vi "Boolean Triggers.vi"() -> ()   [LabVIEW 2019]
panel:
  out "Intake":bool
  out "Trigger":bool
  in  "Joystick for Intake":bool
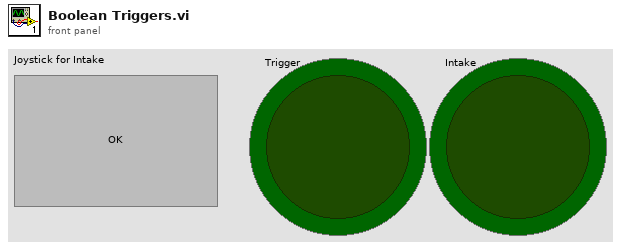
[diagram p1: front panel]
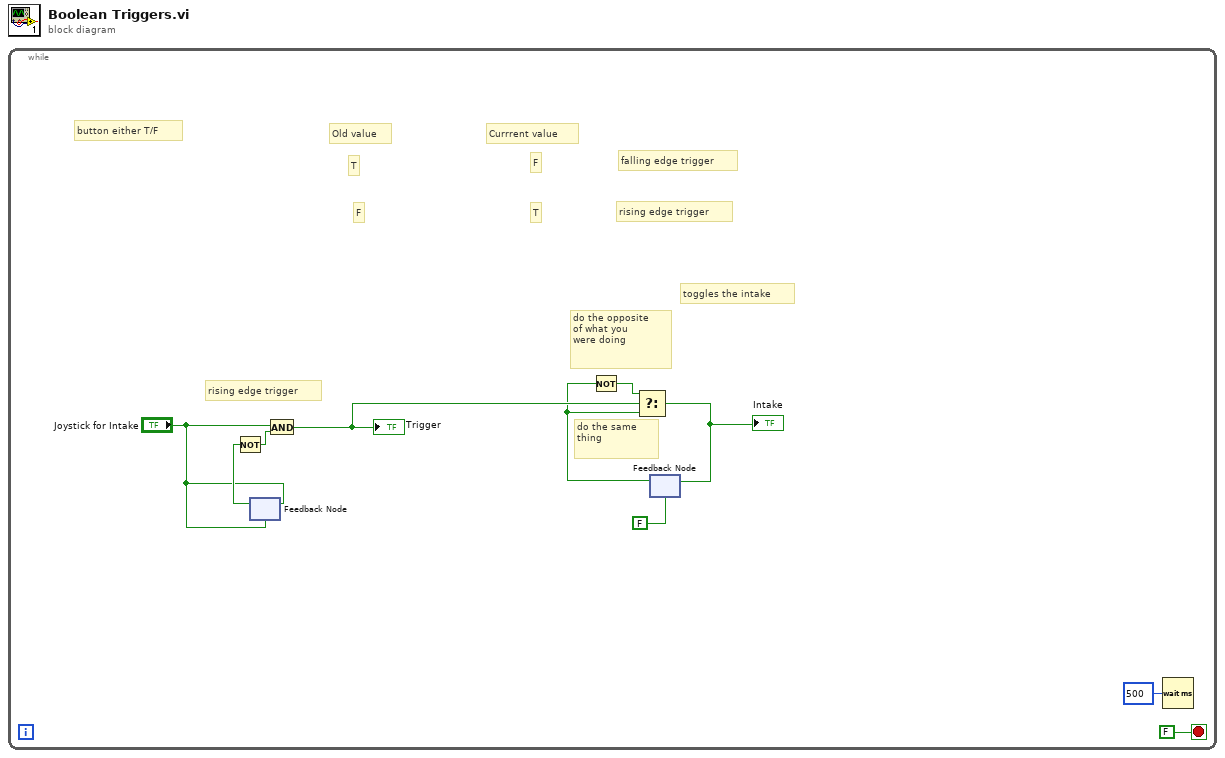
[diagram p0: block diagram]
diagram:
  n1 = while {
    stop <- FALSE stop-if-true
    # "do the opposite\nof what you \nwere doing"
    # "do the same \nthing"
    # "toggles the intake"
    # "rising edge trigger"
    # "rising edge trigger"
    # "T"
    # "F"
    # "falling edge trigger"
    # "T"
    # "F"
    # "Currrent value"
    # "button either T/F"
    # "Old value"
    n2 = feedback-in #1("Joystick for Intake") -> ()
    n3 = feedback #1("Joystick for Intake") -> (w8:bool)
    n4 = Not(x=w8) -> (.not. x?=w6:bool)
    n5 = And(x="Joystick for Intake", y=w6) -> (x .and. y?=w3:bool)
    "Trigger" <- w3
    n6 = feedback #2(FALSE) -> (w1:bool)
    n7 = Not(x=w1) -> (.not. x?=w2:bool)
    n8 = Select(t=w2, s=w3, f=w1) -> (s? t:f=w4:bool)
    "Intake" <- w4
    n9 = feedback-in #2(w4) -> ()
    n10 = Wait (ms)(milliseconds to wait=u32 500) -> ()  [unwired: 1 out]
  }
